vi "Drop Event into subVI.vi"(9 "Current Selection.VI Ref":refnum<vi>, 10 "Target":refnum<vi>, 11 "App Ref":refnum<vi>) -> (0 "error out":errorcluster)   [LabVIEW 2019, in "Panther Dashboard.lvlib"]
uses:
  Panther Dashboard.lvlib
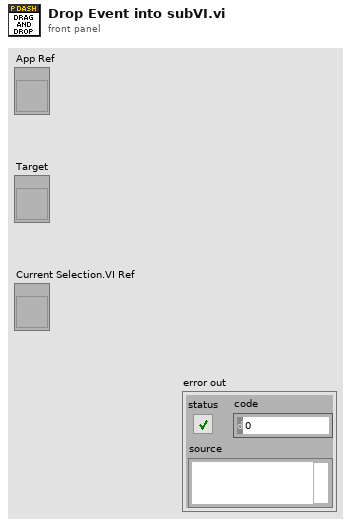
[diagram p1: front panel]
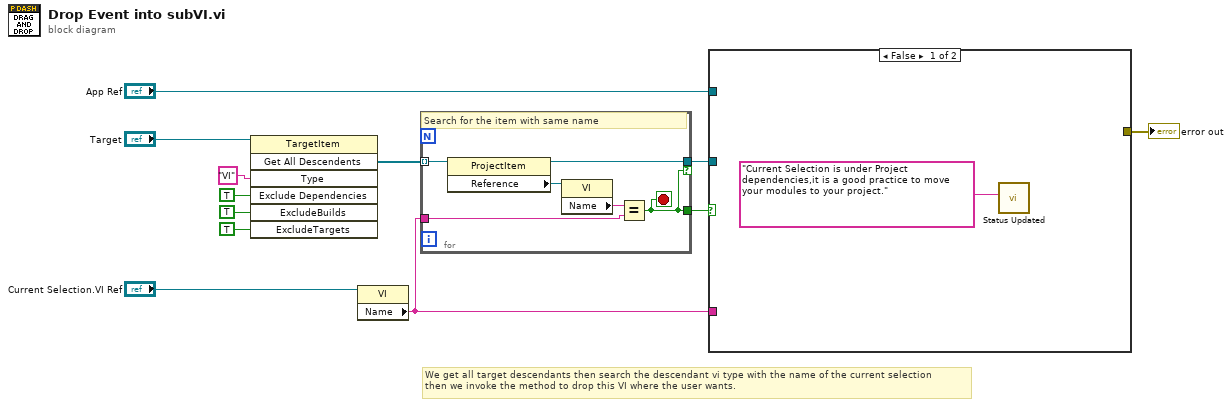
[diagram p0: block diagram]
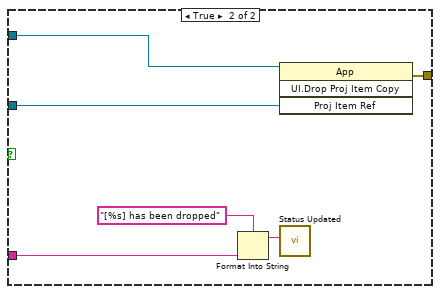
[diagram p2: hidden frame]
diagram:
  # "We get all target descendants then search the descendant vi type with the name of the current selection\nthen we invoke the method to drop this VI where the user wants."
  n1 = invoke class="TargetItem" method="Get All Descendents"(reference="Target", "Type"="VI", "Exclude Dependencies"=TRUE ("ExcludeDependencies"), "ExcludeBuilds"=TRUE, "ExcludeTargets"=TRUE) -> ("All Descendents"=w10:refnum<vi>[])  [unwired: 2 in, 6 out]
  n2 = property class="VI"(reference="Current Selection.VI Ref") -> ("Name"=w1:string)  [unwired: 1 in, 2 out]
  n3 = for {
    tunnel: w10 -> [w17] mode=indexing
    tunnel: [w16] -> w9 if=w18
    tunnel: [w18] -> w8
    tunnel: w1 -> [w14]
    stop <- w18 stop-if-true
    # "Search for the item with same name"
    n4 = property class="ProjectItem"(reference=w17) -> (reference out=w16:refnum<vi>, "Reference"=w15:refnum<vi>)  [unwired: 1 in, 1 out]
    n5 = property class="VI"(reference=w15) -> ("Name"=w13:string)  [unwired: 1 in, 2 out]
    n6 = Equal?(x=w13, y=w14) -> (x = y?=w18:bool)
  }
  n7 = case shown="False" w8 {
    tunnel: "App Ref" -> [_ w24]
    tunnel: [_ w25] -> w12
    tunnel: w9 -> [_ w23]
    tunnel: w1 -> [_ w21]
    frame False {
      n8 = call "Status Updated.vi"("Status"="Current Selection is under Project dependencies,it is a good practice to move your modules to your project." ("format string")) -> ()  [unwired: 10 in, 1 out]
    }
    frame True {
      n9 = Format Into String(format string="[%s] has been dropped", w21) -> (resulting string=w22:string)  [unwired: 2 in, 1 out]
      n10 = invoke class="App" method="UI.Drop Proj Item Copy"(reference=w24, "Proj Item Ref"=w23) -> (error out=w25:errorcluster)  [unwired: 2 in, 3 out]
      n11 = call "Status Updated.vi"("Status"=w22) -> ()  [unwired: 10 in, 1 out]
    }
  }
  "error out" <- w12
